vi "Analog_IP_Data.vi"(7 "Refnum in":refnum<k21>, 8 "error in (no error)":errorcluster, 9 "Constants LL":T1, 10 "Use ATI":bool) -> (0 "Tared FT Reading":dbl[](array[numeric]), 1 "Tension Sensors Data":dbl[](array[numeric]), 2 "Refnum out":refnum<k21>, 3 "ATI Sensor Data":dbl[](array[numeric]), 4 "Toe":dbl format="%0.2f", 5 "error out":errorcluster, 6 "Heel":dbl format="%0.2f", 11 "Vicon Sync":dbl format="%0.2f")   [LabVIEW 2024]
uses:
  typeDef/constants_LL.ctl
  <vilib>/Analysis/3filter.llb/Filter Passband Type.ctl
  <vilib>/DAQmx/read.llb/DAQmx Read (Analog 2D DBL NChan NSamp).vi
  <vilib>/Analysis/baseanly.llb/Mean (DBL).vi
  <vilib>/Analysis/baseanly.llb/A x Vector.vi
  <vilib>/DAQmx/miscellaneous.llb/DAQmx Fill In Error Info.vi
  <vilib>/ptbypt/NI_PtbyPt.lvlib
  <vilib>/Analysis/NI_AALBase.lvlib
panel:
  out "Array":dbl[](array[numeric])
  out "appended array":dbl[](array[numeric])
  in  "taresensors":bool
  out "A x Vector 3":dbl[](array[numeric]) format="%.2f"
  out "Tared FT Reading 2":dbl[](array[numeric])
  in  "Tare 2":bool
  out "A x Vector 2":dbl[](array[numeric]) format="%.2f"
  in  "Tare":bool
  out "A x Vector":dbl[](array[numeric]) format="%.2f"
  in  "Initialize":bool
  out "Filtered x":dbl format="%0.2f"
  out "Waveform Chart 2":dbl[](graph)
  out "Waveform Chart":dbl[](graph)
  # "-0.1"
  # "4.63"
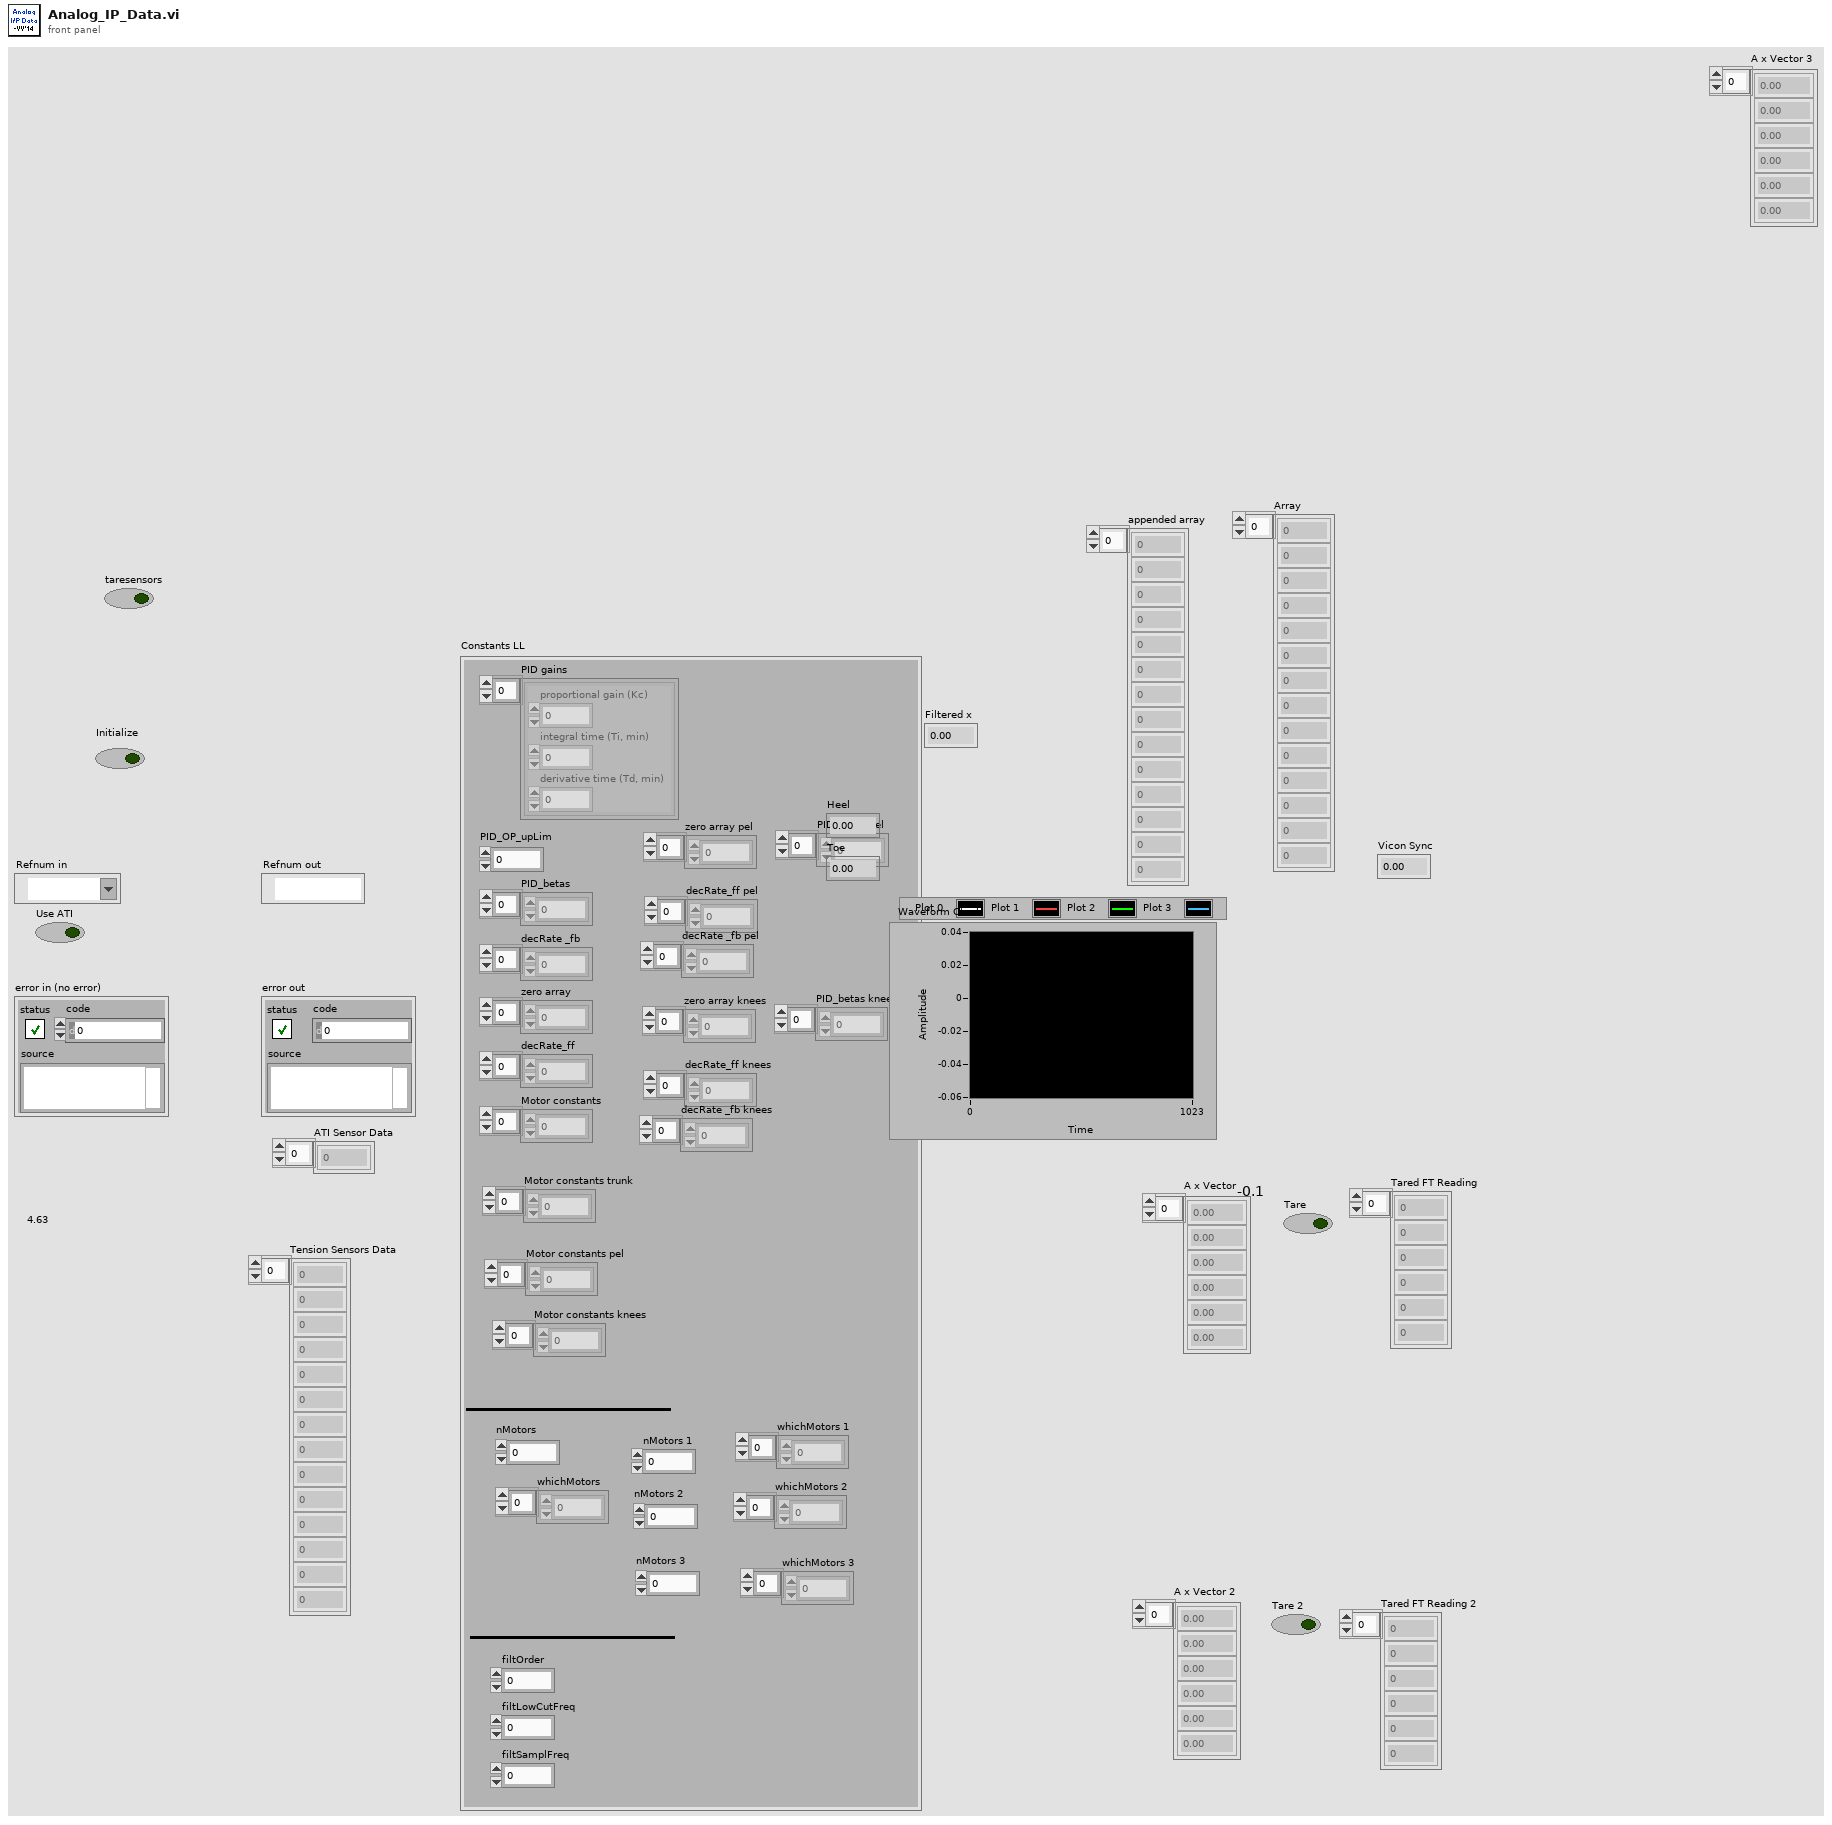
[diagram p1: front panel]
types:
  T1 = typedef "constants_LL.ctl" = cluster{"zero array":dbl[], "decRate_ff":dbl[], "Motor constants":dbl[], "PID gains":cluster{"proportional gain (Kc)":dbl, "integral time (Ti, min)":dbl, "derivative time (Td, min)":dbl}[], "decRate _fb":dbl[], "PID_OP_upLim":dbl, "nMotors":i32, "PID_betas":dbl[], "filtOrder":i32, "filtLowCutFreq":dbl, "filtSamplFreq":dbl, "whichMotors":i32[], "nMotors 1":i32, "nMotors 2":i32, "Motor constants pel":dbl[], "Motor constants trunk":dbl[], "whichMotors 1":i32[], "whichMotors 2":i32[], "zero array pel":dbl[], "decRate_ff pel":dbl[], "decRate _fb pel":dbl[], "PID_betas pel":dbl[], "whichMotors 3":i32[], "nMotors 3":i32, "Motor constants knees":dbl[], "zero array knees":dbl[], "decRate_ff knees":dbl[], "decRate _fb knees":dbl[], "PID_betas knees":dbl[]}
  T2 = typedef "NI_AALBase.lvlib/Filter Passband Type.ctl" = enum32{"Lowpass", "Highpass", "Bandpass", "Bandstop"}
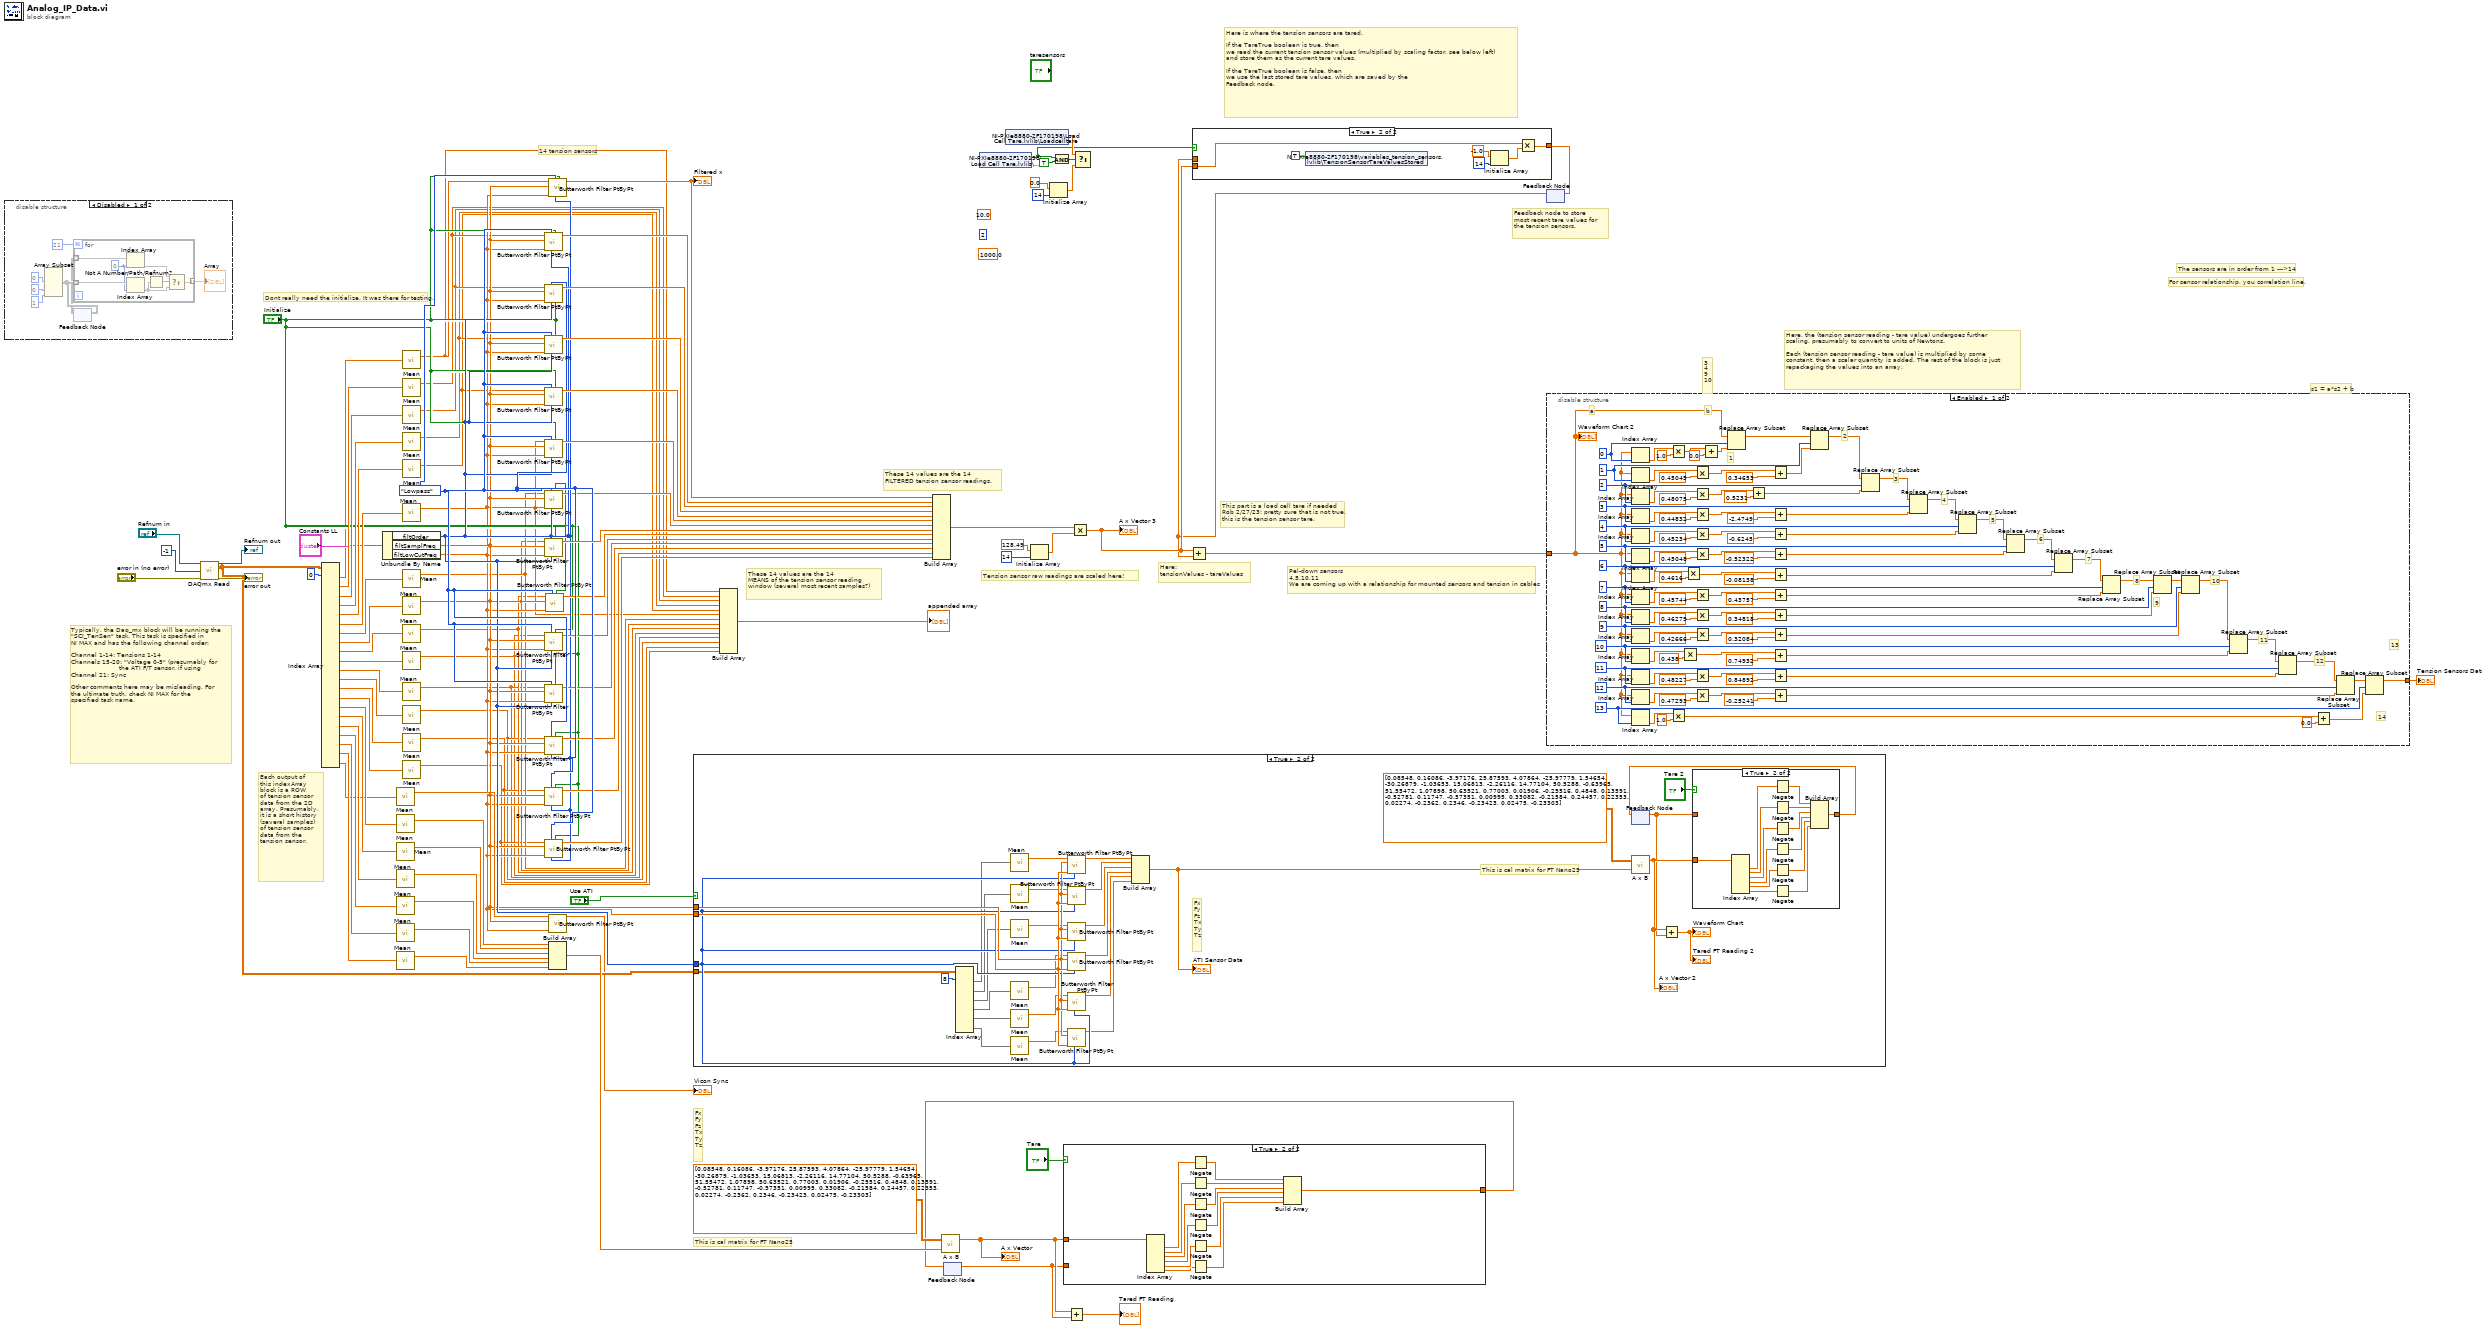
[diagram p0: block diagram]
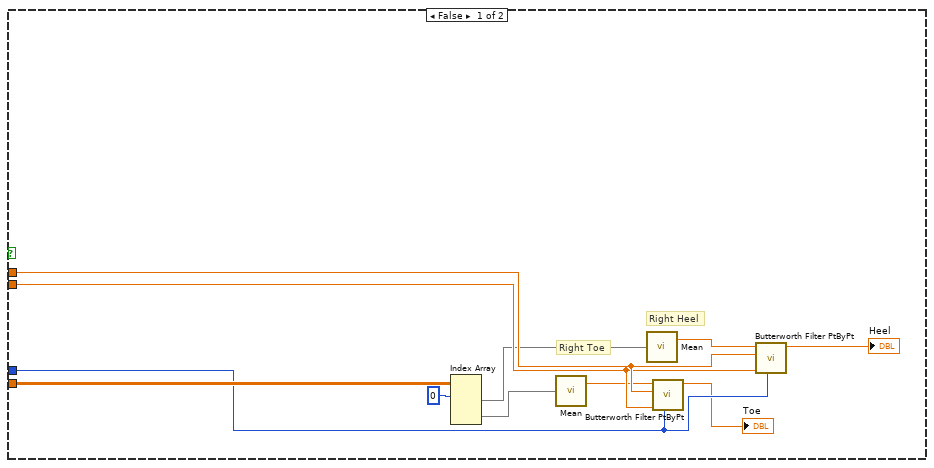
[diagram p6: hidden frame]
diagram:
  w64 = Filter_Passband_Type."Lowpass" ("filter type")
  (unwired) 2 ("order")
  (unwired) 10.0 ("low cutoff freq: fl")
  (unwired) 1000.0 ("sampling freq: fs")
  # "Here, the (tension sensor reading - tare value) undergoes further \nscaling, presumably to convert to units of Newtons. \n\nEach (tension sensor reading - tare value) is multiplied by some \nconstant, then a scalar quantity is added. The rest of the block is just \nrepackaging the values into an array."
  # "Here: \ntensionValues - tareValues"
  # "Each output of \nthis indexArray \nblock is a ROW\nof tension sensor\ndata from the 2D\narray. Presumably,\nit is a short history\n(several samples)\nof tension sensor \ndata from the \ntension sensor."
  # "These 14 values are the 14\nMEANS of the tension sensor reading\nwindow (several most recent samples?)"
  # "Typically, the Daq_mx block will be running the \n\"SCI_TenSen\" task. This task is specified in \nNI MAX and has the following channel order:\n\nChannel 1-14: Tensions 1-14\nChannels 15-20: \"Voltage 0-5\" (presumably for\n                        the ATI F/T sensor, if using\nChannel 21: Sync\n\nOther comments here may be misleading. For \nthe ultimate truth, check NI MAX for the  \nspecified task name."
  # "These 14 values are the 14\nFILTERED tension sensor readings."
  # "Tension sensor raw readings are scaled here!"
  # "Feedback node to store \nmost recent tare values for \nthe tension sensors."
  # "Here is where the tension sensors are tared. \n\nIf the TareTrue boolean is true, then \nwe read the current tension sensor values (multiplied by scaling factor, see below left)\nand store them as the current tare values. \n\nIf the TareTrue boolean is false, then \nwe use the last stored tare values, which are saved by the\nFeedback node."
  # "The sensors are in order from 1 --->14"
  # "For sensor relationship, you correlation line."
  # "3\n4\n9\n10"
  # "s1 = a*s2 + b"
  # "Pel-down sensors\n4,5,10,11\nWe are coming up with a relationship for mounted sensors and tension in cables"
  # "This is cal matrix for FT Nano25"
  # "Fx\nFy\nFz\nTx\nTy\nTz"
  # "This part is a load cell tare if needed\nRob 2/27/23: pretty sure that is not true,\nthis is the tension sensor tare."
  # "Dont really need the initialize. It was there for testing."
  # "14 tension sensors"
  n1 = disable-structure shown="Disabled" {
    frame Disabled {
      n2 = Array Subset(index (row)=0 ("index"), index (col)=0 ("index"), length (col)=1 ("length")) -> (w98:void[][])  [unwired: 2 in]
      n3 = feedback #1() -> (w97:void[][])  [unwired: 1 in]
      n4 = for {
        N: 21 -> [_]
        tunnel: w98 -> [w109] mode=indexing
        tunnel: w97 -> [w106] mode=indexing
        tunnel: [w103] -> w96 mode=indexing
        w105 = 0 ("index")
        n5 = Index Array(array=w106, index=w105) -> (element=w104)
        n6 = Index Array(array=w109, index=w105) -> (element=w107)
        n7 = Not A Number/Path/Refnum?(number/path/refnum=w107) -> (NaN/Path/Refnum?=w108:bool)
        n8 = Select(t=w104, s=w108, f=w107) -> (s? t:f=w103:dbl)
      }
      "Array" <- w96
      n9 = feedback-in #1(w98) -> ()
    }
    frame Enabled {
    }
  }
  n10 = call-poly <vilib>:"DAQmx Read.vi"("task/channels in"="Refnum in", "number of samples per channel"=-1, "error in"="error in (no error)") -> ("task out"=→"Refnum out":refnum<k21>, "data"=w4:dbl[][], "error out"=→"error out":errorcluster)  [unwired: 10 in]
  n11 = Index Array(array=w4, index (row) #1=0 ("index (row)")) -> (element #1=w5:dbl[], element #2=w92:dbl[], element #3=w91:dbl[], element #4=w90:dbl[], element #5=w89:dbl[], element #6=w88:dbl[], element #7=w87:dbl[], element #8=w84:dbl[], element #9=w70:dbl[], element #10=w69:dbl[], element #11=w68:dbl[], element #12=w67:dbl[], element #13=w66:dbl[], element #14=w65:dbl[], element #15=w48:dbl[], element #16=w47:dbl[], element #17=w46:dbl[], element #18=w45:dbl[], element #19=w44:dbl[], element #20=w43:dbl[], element #21=w25:dbl[])  [unwired: 41 in]
  n12 = Unbundle By Name("Constants LL") -> ("filtOrder"=w57:i32, "filtSamplFreq"=w23:dbl, "filtLowCutFreq"=w22:dbl)
  n13 = call-poly <vilib>:"Mean.vi"("X"=w25) -> ("mean"=w24:dbl)  [unwired: 1 out]
  n14 = call-poly <vilib>:"Mean.vi"("X"=w48) -> ("mean"=w42:dbl)  [unwired: 1 out]
  n15 = call-poly <vilib>:"Mean.vi"("X"=w47) -> ("mean"=w41:dbl)  [unwired: 1 out]
  n16 = call-poly <vilib>:"Mean.vi"("X"=w46) -> ("mean"=w40:dbl)  [unwired: 1 out]
  n17 = call-poly <vilib>:"Mean.vi"("X"=w45) -> ("mean"=w39:dbl)  [unwired: 1 out]
  n18 = call-poly <vilib>:"Mean.vi"("X"=w44) -> ("mean"=w38:dbl)  [unwired: 1 out]
  n19 = call-poly <vilib>:"Mean.vi"("X"=w43) -> ("mean"=w37:dbl)  [unwired: 1 out]
  n20 = call-poly <vilib>:"Mean.vi"("X"=w5) -> ("mean"=w21:dbl)  [unwired: 1 out]
  n21 = call-poly <vilib>:"Mean.vi"("X"=w92) -> ("mean"=w20:dbl)  [unwired: 1 out]
  n22 = call-poly <vilib>:"Mean.vi"("X"=w91) -> ("mean"=w19:dbl)  [unwired: 1 out]
  n23 = call-poly <vilib>:"Mean.vi"("X"=w90) -> ("mean"=w18:dbl)  [unwired: 1 out]
  n24 = call-poly <vilib>:"Mean.vi"("X"=w89) -> ("mean"=w17:dbl)  [unwired: 1 out]
  n25 = call-poly <vilib>:"Mean.vi"("X"=w88) -> ("mean"=w16:dbl)  [unwired: 1 out]
  n26 = call-poly <vilib>:"Mean.vi"("X"=w87) -> ("mean"=w15:dbl)  [unwired: 1 out]
  n27 = call-poly <vilib>:"Mean.vi"("X"=w84) -> ("mean"=w14:dbl)  [unwired: 1 out]
  n28 = call-poly <vilib>:"Mean.vi"("X"=w70) -> ("mean"=w13:dbl)  [unwired: 1 out]
  n29 = call-poly <vilib>:"Mean.vi"("X"=w69) -> ("mean"=w8:dbl)  [unwired: 1 out]
  n30 = call-poly <vilib>:"Mean.vi"("X"=w68) -> ("mean"=w9:dbl)  [unwired: 1 out]
  n31 = call-poly <vilib>:"Mean.vi"("X"=w67) -> ("mean"=w10:dbl)  [unwired: 1 out]
  n32 = call-poly <vilib>:"Mean.vi"("X"=w66) -> ("mean"=w11:dbl)  [unwired: 1 out]
  n33 = call-poly <vilib>:"Mean.vi"("X"=w65) -> ("mean"=w12:dbl)  [unwired: 1 out]
  n34 = call <vilib>:"Butterworth Filter PtByPt.vi"("initialize"="Initialize", "order"=w57, "filter type"=w64, "low cutoff freq: fl"=w22, "sampling freq: fs"=w23, "x"=w20) -> ("Filtered x"=w71:dbl)  [unwired: 3 in, 1 out]
  n35 = call <vilib>:"Butterworth Filter PtByPt.vi"("initialize"="Initialize", "order"=w57, "filter type"=w64, "low cutoff freq: fl"=w22, "sampling freq: fs"=w23, "x"=w19) -> ("Filtered x"=w73:dbl)  [unwired: 3 in, 1 out]
  n36 = call <vilib>:"Butterworth Filter PtByPt.vi"("initialize"="Initialize", "order"=w57, "filter type"=w64, "low cutoff freq: fl"=w22, "sampling freq: fs"=w23, "x"=w18) -> ("Filtered x"=w72:dbl)  [unwired: 3 in, 1 out]
  n37 = call <vilib>:"Butterworth Filter PtByPt.vi"("initialize"="Initialize", "order"=w57, "filter type"=w64, "low cutoff freq: fl"=w22, "sampling freq: fs"=w23, "x"=w17) -> ("Filtered x"=w74:dbl)  [unwired: 3 in, 1 out]
  n38 = call <vilib>:"Butterworth Filter PtByPt.vi"("initialize"="Initialize", "order"=w57, "filter type"=w64, "low cutoff freq: fl"=w22, "sampling freq: fs"=w23, "x"=w16) -> ("Filtered x"=w75:dbl)  [unwired: 3 in, 1 out]
  n39 = call <vilib>:"Butterworth Filter PtByPt.vi"("initialize"="Initialize", "order"=w57, "filter type"=w64, "low cutoff freq: fl"=w22, "sampling freq: fs"=w23, "x"=w15) -> ("Filtered x"=w56:dbl)  [unwired: 3 in, 1 out]
  n40 = call <vilib>:"Butterworth Filter PtByPt.vi"("initialize"="Initialize", "order"=w57, "filter type"=w64, "low cutoff freq: fl"=w22, "sampling freq: fs"=w23, "x"=w14) -> ("Filtered x"=w76:dbl)  [unwired: 3 in, 1 out]
  n41 = call <vilib>:"Butterworth Filter PtByPt.vi"("initialize"="Initialize", "order"=w57, "filter type"=w64, "low cutoff freq: fl"=w22, "sampling freq: fs"=w23, "x"=w8) -> ("Filtered x"=w62:dbl)  [unwired: 3 in, 1 out]
  n42 = call <vilib>:"Butterworth Filter PtByPt.vi"("initialize"="Initialize", "order"=w57, "filter type"=w64, "low cutoff freq: fl"=w22, "sampling freq: fs"=w23, "x"=w9) -> ("Filtered x"=w61:dbl)  [unwired: 3 in, 1 out]
  n43 = call <vilib>:"Butterworth Filter PtByPt.vi"("initialize"="Initialize", "order"=w57, "filter type"=w64, "low cutoff freq: fl"=w22, "sampling freq: fs"=w23, "x"=w10) -> ("Filtered x"=w60:dbl)  [unwired: 3 in, 1 out]
  n44 = call <vilib>:"Butterworth Filter PtByPt.vi"("initialize"="Initialize", "order"=w57, "filter type"=w64, "low cutoff freq: fl"=w22, "sampling freq: fs"=w23, "x"=w11) -> ("Filtered x"=w59:dbl)  [unwired: 3 in, 1 out]
  n45 = call <vilib>:"Butterworth Filter PtByPt.vi"("initialize"="Initialize", "order"=w57, "filter type"=w64, "low cutoff freq: fl"=w22, "sampling freq: fs"=w23, "x"=w12) -> ("Filtered x"=w58:dbl)  [unwired: 3 in, 1 out]
  n46 = call <vilib>:"Butterworth Filter PtByPt.vi"("initialize"="Initialize", "filter type"=w64, "low cutoff freq: fl"=w22, "sampling freq: fs"=w23, "x"=w13) -> ("Filtered x"=w63:dbl)  [unwired: 4 in, 1 out]
  n47 = call <vilib>:"Butterworth Filter PtByPt.vi"("initialize"="Initialize", "order"=w57, "filter type"=w64, "low cutoff freq: fl"=w22, "sampling freq: fs"=w23, "x"=w21) -> ("Filtered x"=w77:dbl)  [unwired: 3 in, 1 out]
  "Filtered x" <- w77
  n48 = call <vilib>:"Butterworth Filter PtByPt.vi"("low cutoff freq: fl"=w22, "sampling freq: fs"=w23, "x"=w24) -> ("Filtered x"=→"Vicon Sync":dbl)  [unwired: 6 in, 1 out]
  n49 = Build Array(w42, w41, w40, w39, w38, w37) -> (w34:dbl[])
  n50 = case shown="True" "Use ATI" {
    tunnel: w22 -> [w117 w150]
    tunnel: w23 -> [w118 w149]
    tunnel: w57 -> [w119 w148]
    tunnel: w4 -> [w120 w128]
    frame False {
      # "Right Toe"
      # "Right Heel"
      n51 = Index Array(array=w120, index (row) #1=0 ("index (row)")) -> (element #1=w113:dbl[], element #2=w112:dbl[])  [unwired: 3 in]
      n52 = call-poly <vilib>:"Mean.vi"("X"=w112) -> ("mean"=w115:dbl)  [unwired: 1 out]
      n53 = call-poly <vilib>:"Mean.vi"("X"=w113) -> ("mean"=w116:dbl)  [unwired: 1 out]
      n54 = call <vilib>:"Butterworth Filter PtByPt.vi"("order"=w119, "low cutoff freq: fl"=w117, "sampling freq: fs"=w118, "x"=w115) -> ("Filtered x"=→"Toe":dbl)  [unwired: 5 in, 1 out]
      n55 = call <vilib>:"Butterworth Filter PtByPt.vi"("order"=w119, "low cutoff freq: fl"=w117, "sampling freq: fs"=w118, "x"=w116) -> ("Filtered x"=→"Heel":dbl)  [unwired: 5 in, 1 out]
    }
    frame True {
      # "This is cal matrix for FT Nano25"
      # "Fx\nFy\nFz\nTx\nTy\nTz"
      n56 = Index Array(array=w128, index (row) #1=8 ("index (row)")) -> (element #1=w134:dbl[], element #2=w133:dbl[], element #3=w132:dbl[], element #4=w131:dbl[], element #5=w130:dbl[], element #6=w129:dbl[])  [unwired: 11 in]
      n57 = call-poly <vilib>:"Mean.vi"("X"=w134) -> ("mean"=w147:dbl)  [unwired: 1 out]
      n58 = call-poly <vilib>:"Mean.vi"("X"=w133) -> ("mean"=w146:dbl)  [unwired: 1 out]
      n59 = call-poly <vilib>:"Mean.vi"("X"=w132) -> ("mean"=w145:dbl)  [unwired: 1 out]
      n60 = call-poly <vilib>:"Mean.vi"("X"=w131) -> ("mean"=w144:dbl)  [unwired: 1 out]
      n61 = call-poly <vilib>:"Mean.vi"("X"=w130) -> ("mean"=w143:dbl)  [unwired: 1 out]
      n62 = call-poly <vilib>:"Mean.vi"("X"=w129) -> ("mean"=w142:dbl)  [unwired: 1 out]
      n63 = call <vilib>:"Butterworth Filter PtByPt.vi"("order"=w148, "low cutoff freq: fl"=w150, "sampling freq: fs"=w149, "x"=w147) -> ("Filtered x"=w141:dbl)  [unwired: 5 in, 1 out]
      n64 = call <vilib>:"Butterworth Filter PtByPt.vi"("order"=w148, "low cutoff freq: fl"=w150, "sampling freq: fs"=w149, "x"=w146) -> ("Filtered x"=w140:dbl)  [unwired: 5 in, 1 out]
      n65 = call <vilib>:"Butterworth Filter PtByPt.vi"("order"=w148, "low cutoff freq: fl"=w150, "sampling freq: fs"=w149, "x"=w145) -> ("Filtered x"=w139:dbl)  [unwired: 5 in, 1 out]
      n66 = call <vilib>:"Butterworth Filter PtByPt.vi"("order"=w148, "low cutoff freq: fl"=w150, "sampling freq: fs"=w149, "x"=w144) -> ("Filtered x"=w138:dbl)  [unwired: 5 in, 1 out]
      n67 = call <vilib>:"Butterworth Filter PtByPt.vi"("order"=w148, "low cutoff freq: fl"=w150, "sampling freq: fs"=w149, "x"=w143) -> ("Filtered x"=w137:dbl)  [unwired: 5 in, 1 out]
      n68 = call <vilib>:"Butterworth Filter PtByPt.vi"("order"=w148, "low cutoff freq: fl"=w150, "sampling freq: fs"=w149, "x"=w142) -> ("Filtered x"=w136:dbl)  [unwired: 5 in, 1 out]
      n69 = Build Array(w141, w140, w139, w138, w137, w136) -> (w122:dbl[])
      "ATI Sensor Data" <- w122
      n70 = feedback #2() -> (w123:dbl[])  [unwired: 1 in]
      n71 = call-poly <vilib>:"A x B.vi"("Vector"=w122, "A"=dbl[][] [[0.08548, 0.16086, -3.97176, 25.87593, 4.07864, -25.97779], [1.54654, -30.26879, -1.03653, 15.06813, -2.26116, 14.77104], [50.5288, -0.63965, 51.55472, 1.07898, 50.63521, 0.77003], [0.01906, -0.25516, 0.4848, 0.13591, -0.52781, 0.11747], [-0.57351, 0.00995, 0.33082, -0.21584, 0.24457, 0.22353], [0.02274, -0.2362, 0.2346, -0.23423, 0.02475, -0.23303]]) -> ("A x Vector"=w125:dbl[])  [unwired: 1 out]
      "A x Vector 2" <- w125
      n72 = Add ("Add.vi")(x=w125, y=w123) -> (x+y=→"Waveform Chart" →"Tared FT Reading 2":dbl[])
      n73 = case shown="True" "Tare 2" {
        tunnel: w125 -> [_ w153]
        tunnel: [w151 w152] -> w124
        tunnel: w123 -> [w151 _]
        frame False {
        }
        frame True {
          n74 = Index Array(array=w153) -> (element #1=w165:dbl, element #2=w164:dbl, element #3=w163:dbl, element #4=w162:dbl, element #5=w161:dbl, element #6=w160:dbl)  [unwired: 6 in]
          n75 = Negate(x=w165) -> (-x=w159:dbl)
          n76 = Negate(x=w164) -> (-x=w158:dbl)
          n77 = Negate(x=w163) -> (-x=w157:dbl)
          n78 = Negate(x=w162) -> (-x=w156:dbl)
          n79 = Negate(x=w161) -> (-x=w155:dbl)
          n80 = Negate(x=w160) -> (-x=w154:dbl)
          n81 = Build Array(w159, w158, w157, w156, w155, w154) -> (w152:dbl[])
        }
      }
      n82 = feedback-in #2(w124) -> ()
    }
  }
  n83 = Build Array(w21, w20, w19, w18, w17, w16, w15, w14, w13, w8, w9, w10, w11, w12) -> (→"appended array":dbl[])
  n84 = Build Array(w77, w71, w73, w72, w74, w75, w56, w76, w63, w62, w61, w60, w59, w58) -> (w6:dbl[])
  n85 = call-poly <vilib>:"A x B.vi"("Vector"=w34, "A"=dbl[][] [[0.08548, 0.16086, -3.97176, 25.87593, 4.07864, -25.97779], [1.54654, -30.26879, -1.03653, 15.06813, -2.26116, 14.77104], [50.5288, -0.63965, 51.55472, 1.07898, 50.63521, 0.77003], [0.01906, -0.25516, 0.4848, 0.13591, -0.52781, 0.11747], [-0.57351, 0.00995, 0.33082, -0.21584, 0.24457, 0.22353], [0.02274, -0.2362, 0.2346, -0.23423, 0.02475, -0.23303]]) -> ("A x Vector"=w33:dbl[])  [unwired: 1 out]
  "A x Vector" <- w33
  n86 = feedback #3() -> (w30:dbl[])  [unwired: 1 in]
  n87 = shared-variable "NI-PXIe8880-2F170198\\Load Cell Tare.lvlib\\TareTrue"() -> (w1:bool)  [unwired: 1 in, 1 out]
  n88 = shared-variable "NI-PXIe8880-2F170198\\Load Cell Tare.lvlib\\Loadcelltare"() -> (w52:dbl[])  [unwired: 1 in, 1 out]
  n89 = Initialize Array(128.49 ("element"), 14 ("dimension size")) -> (w82:dbl[])
  n90 = Initialize Array(0.0 ("element"), 14 ("dimension size")) -> (w49:dbl[])
  n91 = And(x=w1, y=TRUE) -> (x .and. y?=w54:bool)
  n92 = case shown="True" "Tare" {
    tunnel: w33 -> [_ w168]
    tunnel: [w166 w167] -> w31
    tunnel: w30 -> [w166 _]
    frame False {
    }
    frame True {
      n93 = Index Array(array=w168) -> (element #1=w180:dbl, element #2=w179:dbl, element #3=w178:dbl, element #4=w177:dbl, element #5=w176:dbl, element #6=w175:dbl)  [unwired: 6 in]
      n94 = Negate(x=w180) -> (-x=w174:dbl)
      n95 = Negate(x=w179) -> (-x=w173:dbl)
      n96 = Negate(x=w178) -> (-x=w172:dbl)
      n97 = Negate(x=w177) -> (-x=w171:dbl)
      n98 = Negate(x=w176) -> (-x=w170:dbl)
      n99 = Negate(x=w175) -> (-x=w169:dbl)
      n100 = Build Array(w174, w173, w172, w171, w170, w169) -> (w167:dbl[])
    }
  }
  n101 = feedback-in #3(w31) -> ()
  n102 = Add(x=w33, y=w30) -> (x+y=→"Tared FT Reading":dbl[])
  n103 = Multiply(x=w6, y=w82) -> (x*y=w29:dbl[])
  "A x Vector 3" <- w29
  n104 = Select(t=w52, s=w54, f=w49) -> ()  [unwired: 1 out]
  n105 = feedback #4() -> (w2:dbl[])  [unwired: 1 in]
  n106 = Add ("Add.vi")(x=w29, y=w2) -> (x+y=w27:dbl[])
  n107 = case shown="True" w1 {
    tunnel: w29 -> [_ w184]
    tunnel: [w181 w183] -> w28
    tunnel: w2 -> [w181 _]
    frame False {
    }
    frame True {
      n108 = shared-variable "NI-PXIe8880-2F170198\\variables_tension_sensors.lvlib\\TensionSensorTareValuesStored"(TRUE ("TensionSensorTareValuesStored")) -> ()  [unwired: 1 in, 1 out]
      n109 = Initialize Array(-1.0 ("element"), 14 ("dimension size")) -> (w187:dbl[])
      n110 = Multiply(x=w184, y=w187) -> (x*y=w183:dbl[])
    }
  }
  n111 = feedback-in #4(w28) -> ()
  n112 = disable-structure shown="Enabled" {
    disable-tunnel: w27 -> [w199 _]
    disable-tunnel: [w198 _] -> w26
    frame Enabled {
      w202 = 13 ("index")
      w208 = 12 ("index")
      w214 = 11 ("index")
      w220 = 10 ("index")
      w226 = 9 ("index")
      w232 = 8 ("index")
      w238 = 7 ("index")
      w244 = 6 ("index")
      w250 = 5 ("index")
      w256 = 4 ("index")
      w271 = 3 ("index")
      w272 = 2 ("index")
      w273 = 1 ("index")
      w274 = 0 ("index")
      # "14"
      # "13"
      # "12"
      # "11"
      # "10"
      # "9"
      # "8"
      # "7"
      # "6"
      # "5"
      # "4"
      # "3"
      # "2"
      # "1"
      # "b"
      # "a"
      n113 = Index Array(array=w199, index=w274) -> (element=w263:dbl)
      n114 = Index Array(array=w199, index=w273) -> (element=w262:dbl)
      n115 = Index Array(array=w199, index=w272) -> (element=w261:dbl)
      n116 = Index Array(array=w199, index=w271) -> (element=w260:dbl)
      n117 = Index Array(array=w199, index=w256) -> (element=w254:dbl)
      n118 = Index Array(array=w199, index=w250) -> (element=w248:dbl)
      n119 = Index Array(array=w199, index=w244) -> (element=w242:dbl)
      n120 = Index Array(array=w199, index=w238) -> (element=w236:dbl)
      n121 = Index Array(array=w199, index=w232) -> (element=w230:dbl)
      n122 = Index Array(array=w199, index=w226) -> (element=w224:dbl)
      n123 = Index Array(array=w199, index=w220) -> (element=w218:dbl)
      n124 = Index Array(array=w199, index=w214) -> (element=w212:dbl)
      n125 = Index Array(array=w199, index=w208) -> (element=w206:dbl)
      n126 = Index Array(array=w199, index=w202) -> (element=w200:dbl)
      n127 = Multiply(x=w263, y=1.0) -> (x*y=w285:dbl)
      n128 = Multiply(x=w200, y=1.0) -> (x*y=w204:dbl)
      n129 = Multiply(x=w218, y=0.438) -> (x*y=w222:dbl)
      n130 = Multiply(x=w242, y=0.4616) -> (x*y=w246:dbl)
      n131 = Multiply(x=w262, y=0.45045) -> (x*y=w282:dbl)
      n132 = Multiply(x=w261, y=0.48075) -> (x*y=w279:dbl)
      n133 = Multiply(x=w260, y=0.44832) -> (x*y=w276:dbl)
      n134 = Multiply(x=w254, y=0.45234) -> (x*y=w258:dbl)
      n135 = Multiply(x=w248, y=0.45048) -> (x*y=w252:dbl)
      n136 = Multiply(x=w236, y=0.45744) -> (x*y=w240:dbl)
      n137 = Multiply(x=w230, y=0.46279) -> (x*y=w234:dbl)
      n138 = Multiply(x=w224, y=0.42666) -> (x*y=w228:dbl)
      n139 = Multiply(x=w212, y=0.48227) -> (x*y=w216:dbl)
      n140 = Multiply(x=w206, y=0.47293) -> (x*y=w210:dbl)
      n141 = Add(x=w285, y=0.0) -> (x+y=w267:dbl)
      n142 = Replace Array Subset(array=w199, new element=w267, index=w274) -> (w270:dbl[])
      n143 = Add(x=w279, y=0.5231) -> (x+y=w265:dbl)
      n144 = Add(x=w282, y=0.34653) -> (x+y=w266:dbl)
      n145 = Add(x=w276, y=-2.4749) -> (x+y=w264:dbl)
      n146 = Add(x=w258, y=-0.6245) -> (x+y=w255:dbl)
      n147 = Add(x=w252, y=-0.52322) -> (x+y=w249:dbl)
      n148 = Add(x=w246, y=-0.08138) -> (x+y=w243:dbl)
      n149 = Add(x=w240, y=0.43757) -> (x+y=w237:dbl)
      n150 = Add(x=w234, y=0.34818) -> (x+y=w231:dbl)
      n151 = Add(x=w228, y=0.32084) -> (x+y=w225:dbl)
      n152 = Add(x=w222, y=0.74932) -> (x+y=w219:dbl)
      n153 = Add(x=w216, y=0.84892) -> (x+y=w213:dbl)
      n154 = Add(x=w210, y=-0.25241) -> (x+y=w207:dbl)
      n155 = Replace Array Subset(array=w270, new element=w266, index=w273) -> (w269:dbl[])
      n156 = Replace Array Subset(array=w269, new element=w265, index=w272) -> (w268:dbl[])
      n157 = Replace Array Subset(array=w268, new element=w264, index=w271) -> (w197:dbl[])
      n158 = Replace Array Subset(array=w197, new element=w255, index=w256) -> (w196:dbl[])
      n159 = Replace Array Subset(array=w196, new element=w249, index=w250) -> (w195:dbl[])
      n160 = Replace Array Subset(array=w195, new element=w243, index=w244) -> (w194:dbl[])
      n161 = Replace Array Subset(array=w194, new element=w237, index=w238) -> (w193:dbl[])
      n162 = Replace Array Subset(array=w193, new element=w231, index=w232) -> (w192:dbl[])
      n163 = Replace Array Subset(array=w192, new element=w225, index=w226) -> (w191:dbl[])
      n164 = Replace Array Subset(array=w191, new element=w219, index=w220) -> (w190:dbl[])
      n165 = Replace Array Subset(array=w190, new element=w213, index=w214) -> (w189:dbl[])
      n166 = Add(x=w204, y=0.0) -> (x+y=w201:dbl)
      n167 = Replace Array Subset(array=w189, new element=w207, index=w208) -> (w188:dbl[])
      n168 = Replace Array Subset(array=w188, new element=w201, index=w202) -> (w198:dbl[])
      "Waveform Chart 2" <- w199
    }
    frame Disabled {
    }
  }
  "Tension Sensors Data" <- w26
